vi "Resize DI Command Array.vi"(1 "DI-A Command in":T1[](array[typedef]) {"Default Phase Index" max=7; "Sweep [s]" format="%#_3p"; "Command Sequence"."Phase Index" max=7; "Command Sequence"."Duration [s]" min=0 max=100 format="%#_3p"; "Injections" max=511; "Skip Fire Index" max=7; "Angles"."Phase Index" max=7; "Angles"."Duration [s]" min=0 max=100 format="%#_3p"; "Duration [s]" format="%#_3p"; "Frequency [Hz]" format="%#_3p"}) -> (0 "Array":T1[](array[typedef]) {"Default Phase Index" max=7; "Sweep [s]" format="%#_3p"; "Command Sequence"."Phase Index" max=7; "Command Sequence"."Duration [s]" min=0 max=100 format="%#_3p"; "Injections" max=511; "Skip Fire Index" max=7; "Angles"."Phase Index" max=7; "Angles"."Duration [s]" min=0 max=100 format="%#_3p"; "Duration [s]" format="%#_3p"; "Frequency [Hz]" format="%#_3p"})   [LabVIEW 2015]
uses:
  <vilib>/Powertrain Controls/Device Drivers/DCM/DI/RT/Command.ctl
  <vilib>/Powertrain Controls/Device Drivers/DCM/DI/FPGA/Mode.ctl
  <vilib>/Powertrain Controls/Device Drivers/DCM/Rev0/FPGA/Digital Channel.ctl
  <vilib>/Powertrain Controls/Device Drivers/DCM/DI/RT/Command Sequence.ctl
  <vilib>/Powertrain Controls/Device Drivers/DCM/DI/RT/Angle Control.ctl
  <vilib>/Powertrain Controls/Device Drivers/DCM/DI/RT/DCM - RT - DI.lvlib
  <vilib>/Powertrain Controls/Device Drivers/DCM/DI/FPGA/DCM - FPGA - DI.lvlib
  <vilib>/Powertrain Controls/Device Drivers/DCM/Rev0/FPGA/DCM - FPGA.lvlib
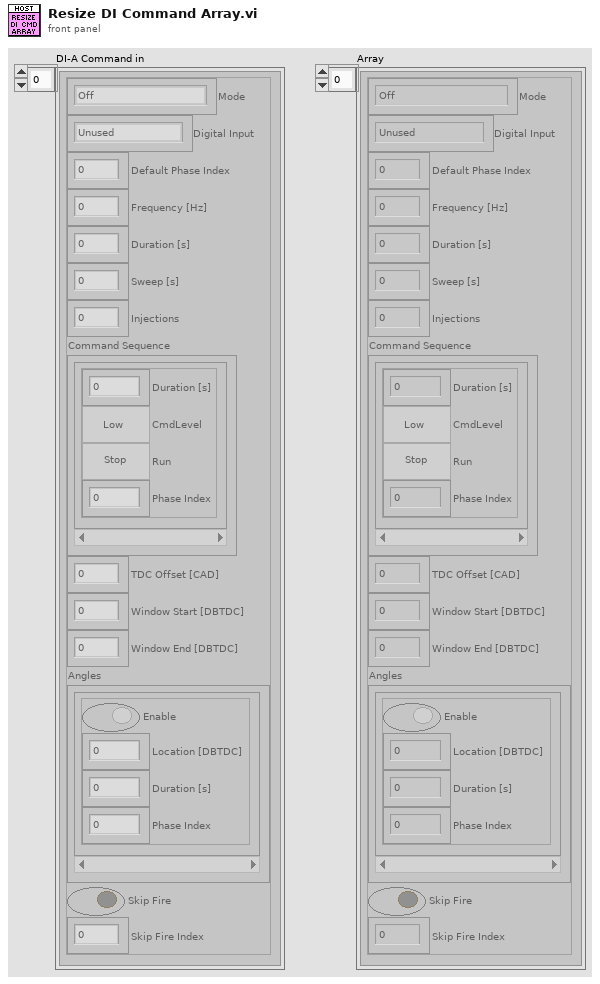
[diagram p1: front panel]
types:
  T1 = typedef "DCM - RT - DI.lvlib/Command.ctl" = cluster{"Mode":T2, "Digital Input":T3, "Default Phase Index":u8, "Frequency [Hz]":sgl, "Duration [s]":sgl, "Sweep [s]":sgl, "Injections":u16, "Command Sequence":T4[], "TDC Offset [CAD]":sgl, "Window Start [DBTDC]":sgl, "Window End [DBTDC]":sgl, "Angles":T5[], "Skip Fire":bool, "Skip Fire Index":u8}
  T2 = typedef "DCM - FPGA - DI.lvlib/Mode.ctl" = enum8{"Off", "Direct", "Calibration", "Triggered Multi-Pulse", "Engine Position Tracking"}
  T3 = typedef "DCM - FPGA.lvlib/Digital Channel.ctl" = enum8{"Unused", "Diff IO 1", "Diff IO 2", "Diff IO 3", "Diff IO 4", "Diff IO 5", "Diff IO 6", "Diff IO 7", "Diff IO 8", "Aux 1", "Aux 2", "Aux 3", "Aux 4", "Aux 5", "Aux 6", "Aux 7", "Aux 8", "User OS"}
  T4 = typedef "DCM - RT - DI.lvlib/Command Sequence.ctl" = cluster{"Duration [s]":sgl, "CmdLevel":bool, "Run":bool, "Phase Index":u8}
  T5 = typedef "DCM - RT - DI.lvlib/Angle Control.ctl" = cluster{"Enable":bool, "Location [DBTDC]":sgl, "Duration [s]":sgl, "Phase Index":u8}
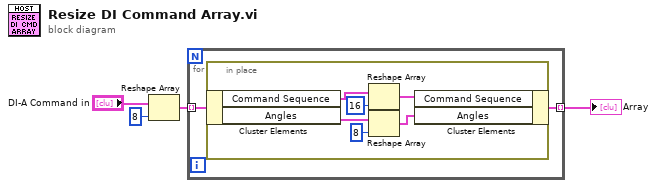
[diagram p0: block diagram]
diagram:
  n1 = Reshape Array("DI-A Command in", 8 ("dimension size")) -> (w1:T1[])
  n2 = for {
    tunnel: w1 -> [w6] mode=indexing
    tunnel: [w5] -> w3 mode=indexing
    n3 = in-place {
      n4 = in-place-cluster #1(w6) -> ("Command Sequence"=w9:T4[], "Angles"=w12:T5[])
      n5 = Reshape Array(w9, 16 ("dimension size")) -> (w8:T4[])
      n6 = Reshape Array(w12, 8 ("dimension size")) -> (w11:T5[])
      n7 = in-place-cluster #1("Command Sequence"=w8, "Angles"=w11) -> (w5:T1)
    }
  }
  "Array" <- w3
